vi "runs.list.vi"(8 "error in":errorcluster, 11 "asset in":refnum<class "asset.lvclass">) -> (0 "error out":errorcluster, 2 "Runs":refnum<class "Run.lvclass">[](array[class]), 3 "asset out":refnum<class "asset.lvclass">)   [LabVIEW 2020, in "asset.lvclass"]
uses:
  asset.lvclass
  Nominal Client/Nominal Client.lvclass
  <vilib>/JDP Science/JSONtext/JSONtext.lvlib
  Run/Run.lvclass
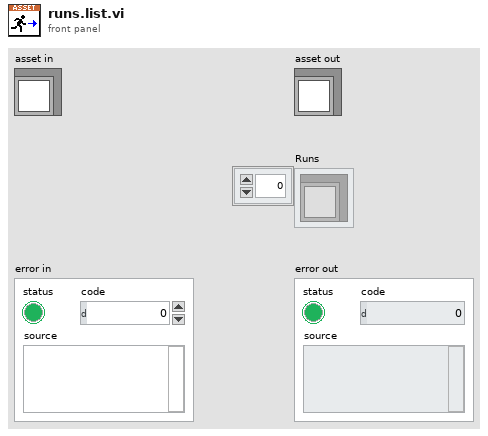
[diagram p1: front panel]
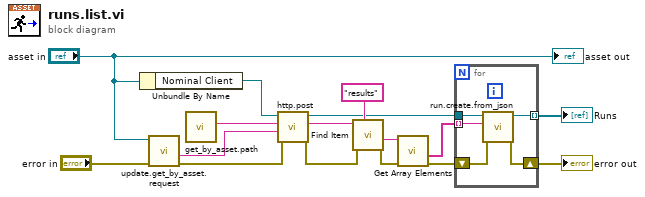
[diagram p0: block diagram]
diagram:
  n1 = Unbundle By Name("asset in") -> ("Nominal Client"=w4:refnum<class "Nominal Client.lvclass">)
  n2 = call "update.get_by_asset.request.vi"("error in"="error in", "asset"="asset in") -> ("error out"=w15:errorcluster, "Request"=w16:string)  [unwired: 8 in]
  n3 = call "get_by_asset.path.vi"() -> ("path"=w14:string)  [unwired: 11 in]
  n4 = call "http.post.vi"("error in"=w15, "Request body"=w16, "Path"=w14, "Nominal Client in"=w4) -> ("error out"=w9:errorcluster, "Response"=w8:string, "Nominal Client out"=w6:refnum<class "Nominal Client.lvclass">)  [unwired: 4 in, 1 out]
  n5 = call <vilib>:"Find Item.vi"("$Path or Item Name"="results", "error in (no error)"=w9, "JSON"=w8) -> ("error out"=w10:errorcluster, "<JSON>"=w7:string)  [unwired: 5 in, 2 out]
  n6 = call <vilib>:"Get Array Elements.vi"("error in (no error)"=w10, "JSON"=w7) -> ("error out"=w11:errorcluster, "<JSON>"=w12:string[])  [unwired: 7 in, 1 out]
  n7 = for {
    tunnel: [w21] -> w3 mode=indexing
    tunnel: w12 -> [w19] mode=indexing
    shift-right: [w20] -> w2
    shift-left: w11 -> [w18]
    tunnel: w6 -> [w17]
    n8 = call "run.create.from_json.vi"("error in"=w18, "JSON"=w19, "Nominal Client"=w17) -> ("error out"=w20:errorcluster, "Run out"=w21:refnum<class "Run.lvclass">)  [unwired: 7 in]
  }
  "error out" <- w2
  "Runs" <- w3
  "asset out" <- "asset in"
